vi "Wait for Acquisition Complete.vi"(8 "error in (no error)":errorcluster, 10 "Maximum Time (10000)":u32=10000, 11 "VISA resource name":refnum<visa-resource-name>) -> (0 "error out":errorcluster, 3 "VISA resource name out":refnum<visa-resource-name>)   [LabVIEW 2019, in "Agilent 2000 3000 X-Series.lvlib"]
doc: "Waits for the current waveform acquisition to finish. This VI should be called after Initiate VI and before Fetch Waveform VI.\n\n<B>Note(s):</B>\nUse this VI only with other low-level VIs. The high-level VIs automatically incorporate this functionality. This VI does not check the instrument status."
uses:
  Agilent 2000 3000 X-Series.lvlib
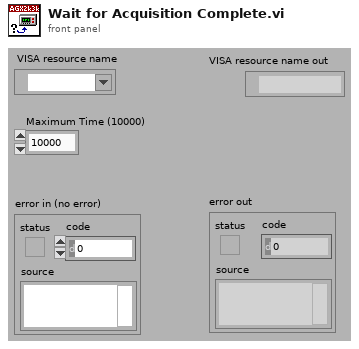
[diagram p1: front panel]
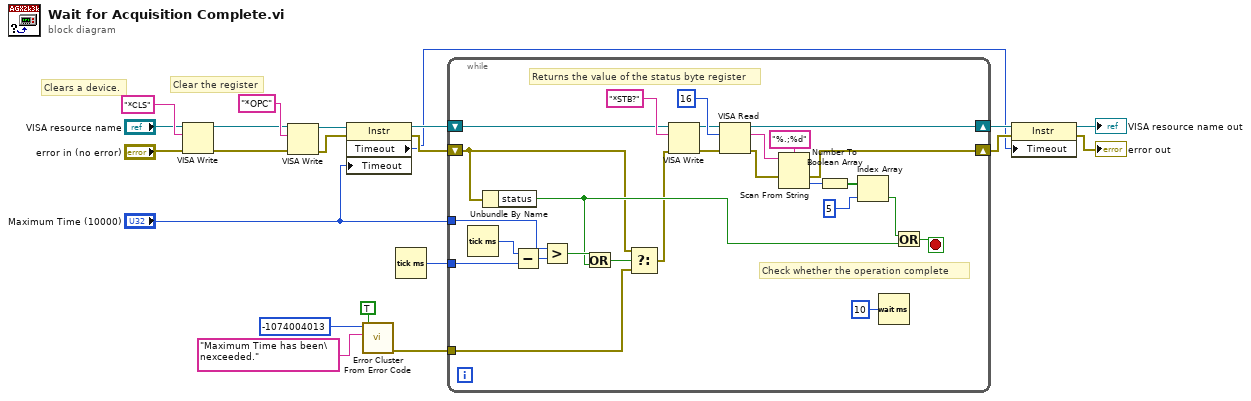
[diagram p0: block diagram]
diagram:
  # "Clears a device."
  # "Clear the register"
  n1 = VISA Write(VISA resource name="VISA resource name", write buffer="*CLS", error in (no error)="error in (no error)") -> (VISA resource name out=w14:refnum<visa-resource-name>, error out=w13:errorcluster)  [unwired: 1 out]
  n2 = VISA Write(VISA resource name=w14, write buffer="*OPC", error in (no error)=w13) -> (VISA resource name out=w6:refnum<visa-resource-name>, error out=w5:errorcluster)  [unwired: 1 out]
  n3 = property class="Instr"(reference=w6, error in=w5, "Timeout"="Maximum Time (10000)") -> (reference out=w4:refnum<visa-resource-name>, error out=w3:errorcluster, "Timeout"=w1:u32)
  n4 = call <vilib>:"Error Cluster From Error Code.vi"("show call chain? (False)"=TRUE, "error message (\"\")"="Maximum Time has been\nexceeded." ("error message (\"\")"), "error code (0)"=-1074004013) -> ("error out"=w16:errorcluster)  [unwired: 1 in, 5 out]
  n5 = Tick Count (ms)() -> (millisecond timer value=w21:u32)
  n6 = while {
    tunnel: "Maximum Time (10000)" -> [w30]
    tunnel: w21 -> [w38]
    tunnel: w16 -> [w25]
    shift-right: [w36] -> w10
    shift-left: w3 -> [w23]
    shift-right: [w45] -> w9
    shift-left: w4 -> [w42]
    stop <- w31 stop-if-true
    # "Check whether the operation complete"
    # "Returns the value of the status byte register"
    n7 = Tick Count (ms)() -> (millisecond timer value=w39:u32)
    n8 = Unbundle By Name(w23) -> ("status"=w26:bool)
    n9 = Subtract(x=w39, y=w38) -> (x-y=w29:u32)
    n10 = Greater?(x=w30, y=w29) -> (0:w28:bool)
    n11 = Or(x=w28, y=w26) -> (x .or. y?=w27:bool)
    n12 = Select(t=w23, s=w27, f=w25) -> (s? t:f=w24:errorcluster)
    n13 = VISA Write(VISA resource name=w42, write buffer="*STB?", error in (no error)=w24) -> (VISA resource name out=w40:refnum<visa-resource-name>, error out=w41:errorcluster)  [unwired: 1 out]
    n14 = VISA Read(VISA resource name=w40, byte count=u32 16, error in (no error)=w41) -> (VISA resource name out=w45:refnum<visa-resource-name>, read buffer=w47:string, error out=w37:errorcluster)  [unwired: 1 out]
    n15 = Scan From String(format string="%.;%d", input string=w47, error in=w37) -> (error out=w36:errorcluster, output 1=w33:i32)  [unwired: 1 in, 3 out]
    n16 = Number To Boolean Array(number=w33) -> (Boolean array=w34:bool[])
    n17 = Index Array(array=w34, index=5) -> (element=w32:bool)
    n18 = Wait (ms)(milliseconds to wait=u32 10) -> ()  [unwired: 1 out]
    n19 = Or(x=w32, y=w26) -> (x .or. y?=w31:bool)
  }
  n20 = property class="Instr"(reference=w9, error in=w10, "Timeout"=w1) -> (reference out=→"VISA resource name out":refnum<visa-resource-name>, error out=→"error out":errorcluster)
